vi "Write Output Terminal.vi"(8 "error in (no error)":errorcluster, 10 "Output Terminal":refnum<vi>, 11 "PainOutputTerminal in":refnum<class "PainOutputTerminal.lvclass">) -> (0 "error out":errorcluster, 3 "PainOutputTerminal out":refnum<class "PainOutputTerminal.lvclass">)   [LabVIEW 2016, in "PainOutputTerminal.lvclass"]
uses:
  PainOutputTerminal.lvclass
  PainOutputTerminal.lvclass/PainOutputTerminal.ctl
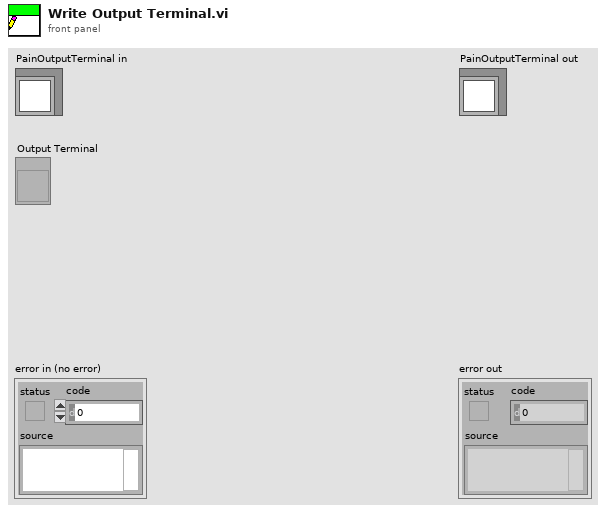
[diagram p1: front panel]
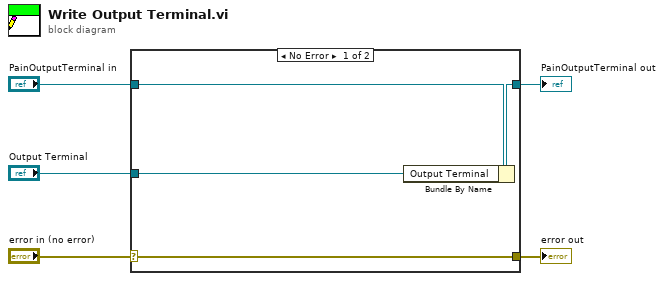
[diagram p0: block diagram]
diagram:
  n1 = case shown="No Error" "error in (no error)" {
    selector: "error in (no error)" -> [w9 w10]
    tunnel: [w9 w10] -> w4
    tunnel: [w7 w11] -> w2
    tunnel: "PainOutputTerminal in" -> [w8 w11]
    tunnel: "Output Terminal" -> [w6 _]
    frame No Error {
      n2 = Bundle By Name(cluster=w8, "Output Terminal"=w6) -> (w7:refnum<class "PainOutputTerminal.lvclass">)
    }
    frame Error {
    }
  }
  "error out" <- w4
  "PainOutputTerminal out" <- w2
